vi "Write Coords.vi"(6 "Coordinates":T1, 11 "Handle Activate Menu On Tree Item Msg in":refnum<class "Handle Activate Menu On Tree Item Msg.lvclass">) -> (3 "Handle Activate Menu On Tree Item Msg out":refnum<class "Handle Activate Menu On Tree Item Msg.lvclass">)   [LabVIEW 2017, in "File Explorer.lvlib" / "Handle Activate Menu On Tree Item Msg.lvclass"]
uses:
  <vilib>/gpm_packages/@cs/file-explorer-extension/Source/File Explorer/File Explorer Messages/Handle Activate Menu On Tree Item Msg/Handle Activate Menu On Tree Item Msg.lvclass
  <vilib>/Utility/miscctls.llb/LVPoint32TypeDef.ctl
  <vilib>/gpm_packages/@cs/file-explorer-extension/Source/File Explorer/File Explorer Messages/Handle Activate Menu On Tree Item Msg/Handle Activate Menu On Tree Item Msg.lvclass/Handle Activate Menu On Tree Item Msg.ctl
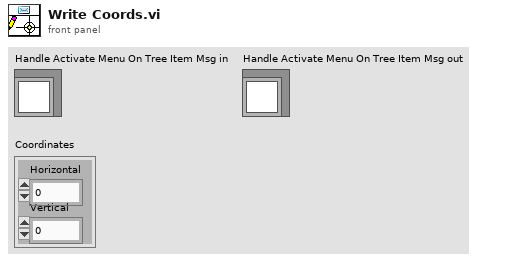
[diagram p1: front panel]
types:
  T1 = typedef "LVPoint32TypeDef.ctl" = cluster{"Horizontal":i32, "Vertical":i32}
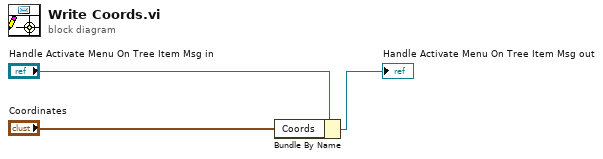
[diagram p0: block diagram]
diagram:
  n1 = Bundle By Name(cluster="Handle Activate Menu On Tree Item Msg in", "Coords"="Coordinates") -> (→"Handle Activate Menu On Tree Item Msg out":refnum<class "Handle Activate Menu On Tree Item Msg.lvclass">)
